vi "Configure Test Executive.vi"(6 "Compatibility Helper Type":refnum<class "ICompatibility Helper.lvclass">, 7 "Show IDs?":bool, 8 "Path Builder Type":refnum<class "IPath Builder.lvclass">, 9 "Test Executive Type":refnum<class "ITest Executive.lvclass">, 10 "Persistence Type":refnum<class "IPersist.lvclass">, 11 "Test Executive Builder Model in":refnum<class "Test Executive Builder Model.lvclass">) -> (3 "Test Executive Builder Model out":refnum<class "Test Executive Builder Model.lvclass">)   [LabVIEW 2017, in "Test Executive Builder Model.lvclass"]
uses:
  Test Executive Builder Model.lvclass
  <vilib>/gpm_packages/@cs/test-executive/Source/Test Executive/ITestExecutive/ITest Executive.lvclass
  <vilib>/gpm_packages/@cs/test-executive/Source/Path Builder/IPath Builder/IPath Builder.lvclass
  <vilib>/gpm_packages/@cs/test-executive/Source/Compatibility Helper/ICompatibility Helper.lvclass
  <vilib>/gpm_packages/@cs/persistence/source/IPersist/IPersist.lvclass
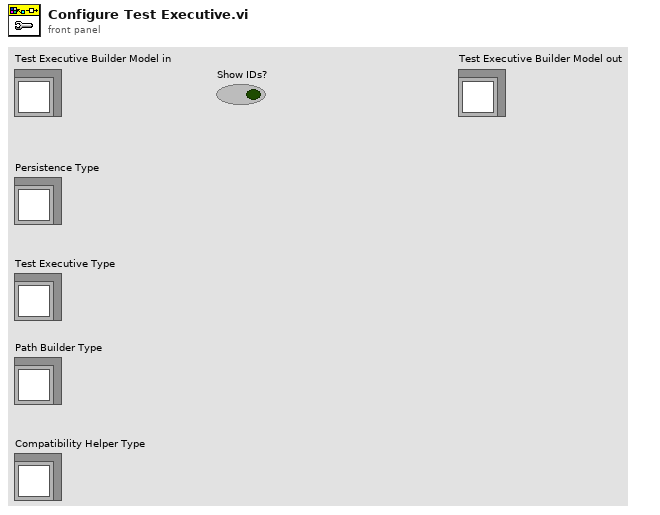
[diagram p1: front panel]
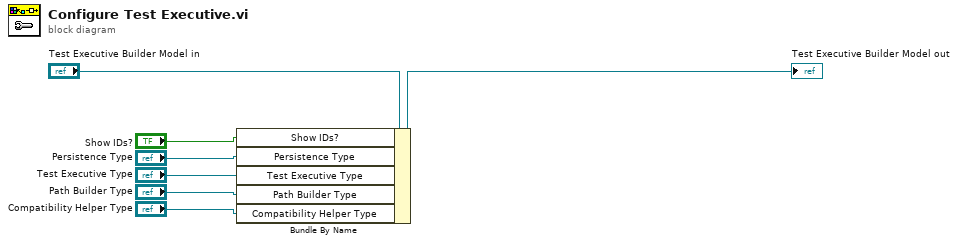
[diagram p0: block diagram]
diagram:
  n1 = Bundle By Name(cluster="Test Executive Builder Model in", "Show IDs?"="Show IDs?", "Persistence Type"="Persistence Type", "Test Executive Type"="Test Executive Type", "Path Builder Type"="Path Builder Type", "Compatibility Helper Type"="Compatibility Helper Type") -> (→"Test Executive Builder Model out":refnum<class "Test Executive Builder Model.lvclass">)
